vi "Conn getData.vi"(4 "error in (no error)":errorcluster, 7 "connection reference":T2) -> (0 "error out":errorcluster, 1 "object is locked?":bool, 2 "data":T1, 3 "connection reference out":T2)   [LabVIEW 2020, in "NI_Database_API.lvlib"]
doc: "Returns the data of a <B>Connection</B> object.\n\nIf the object is currently locked for modification, <B>object is locked?</B> will return TRUE.\n\n[GOOP 1.0/1.0]"
uses:
  <vilib>/addons/database/NI_Database_API.lvlib
  <vilib>/addons/database/Connection.llb/Conn DataMembers.ctl
  <vilib>/addons/database/Connection.llb/Conn ObjectReference.ctl
  <vilib>/Utility/_goopsup.llb/GOOP Object Repository Method.ctl
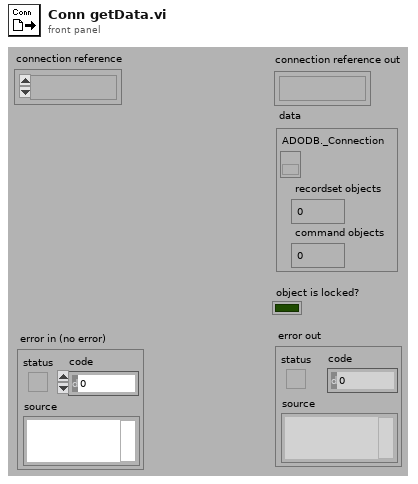
[diagram p1: front panel]
types:
  T1 = typedef "NI_Database_API.lvlib/Conn DataMembers.ctl" = cluster{"ADODB._Connection":refnum<k7>, "recordset objects":i32, "command objects":i32}
  T2 = typedef "NI_Database_API.lvlib/Conn ObjectReference.ctl" = refnum<k1>
  T3 = typedef "GOOP Object Repository Method.ctl" = enum16{"Create", "GetCopy", "GetModify", "Set", "Destroy", "Create Static", "Get All Refs", "Reset", "Get Statistics"}
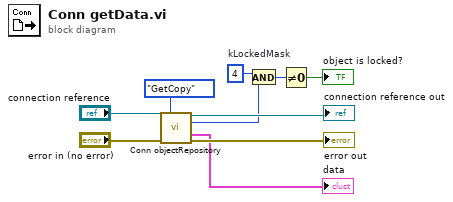
[diagram p0: block diagram]
diagram:
  w3 = 4  # kLockedMask
  n1 = call <vilib>:"Conn objectRepository.vi"("connection reference"="connection reference", "method"=GOOP_Object_Repository_Method."GetCopy", "error in (no error)"="error in (no error)") -> ("connection reference out"=→"connection reference out":T2, "flags out"=w2:i32, "classDataOut"=→"data":T1, "error out"=→"error out":errorcluster)  [unwired: 6 in, 3 out]
  n2 = And(x=w3, y=w2) -> (x .and. y?=w4:i32)
  n3 = Not Equal To 0?(x=w4) -> (x != 0?=→"object is locked?":bool)
